vi "MeasureSystemTime.vi"(8 "error in":errorcluster, 11 "VISA resource name":refnum<visa-resource-name>) -> (0 "error out":errorcluster, 1 "System time end":dbl=437416.625 format="%.3f", 2 "System time start":dbl=437416.625 format="%.3f", 3 "VISA resource name out":refnum<visa-resource-name>)   [LabVIEW 2018, in "GP22_TDC_Arduinoed.lvlib"]
doc: "Gets the system time at the start and end of comms. For use in clock sync via NTP-style algorithm."
uses:
  GP22_TDC_Arduinoed.lvlib
  <vilib>/regexp/Match Regular Expression.xnode
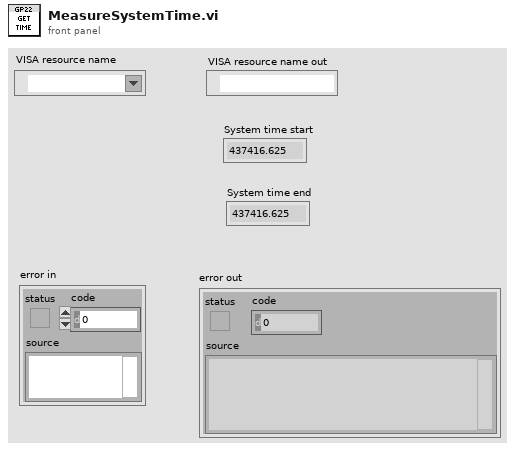
[diagram p1: front panel]
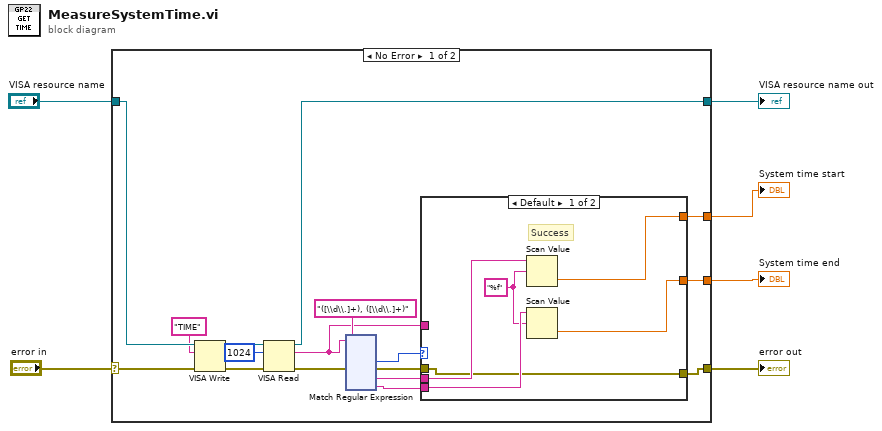
[diagram p0: block diagram]
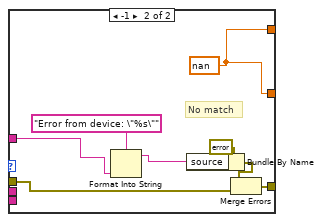
[diagram p2: hidden frame]
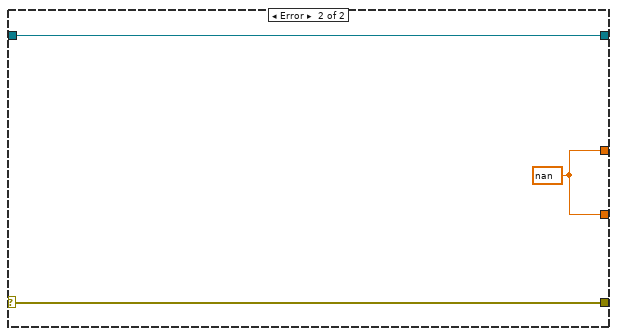
[diagram p3: hidden frame]
diagram:
  n1 = case shown="No Error" "error in" {
    selector: "error in" -> [w23 w157]
    tunnel: [w11 w157] -> w5
    tunnel: [w16 w156] -> w4
    tunnel: "VISA resource name" -> [w22 w156]
    tunnel: [w8 w155] -> w2
    tunnel: [w7 w155] -> w1
    frame No Error {
      n2 = VISA Write(VISA resource name=w22, write buffer="TIME", error in (no error)=w23) -> (VISA resource name out=w19:refnum<visa-resource-name>, error out=w20:errorcluster)  [unwired: 1 out]
      n3 = VISA Read(VISA resource name=w19, byte count=u32 1024, error in (no error)=w20) -> (VISA resource name out=w16:refnum<visa-resource-name>, read buffer=w12:string, error out=w17:errorcluster)  [unwired: 1 out]
      n4 = xnode "Match Regular Expression"("input string"=w12, "regular expression"="([\\d\\.]+), ([\\d\\.]+)", "error in"=w17) -> ("offset past match"=w14:i32, "error out"=w13:errorcluster, "submatch 1"=w10:string, "submatch 2"=w9:string)  [unwired: 3 in, 3 out]
      n5 = case shown="Default" w14 {
        tunnel: w13 -> [w25 w34]
        tunnel: w12 -> [_ w33]
        tunnel: [w25 w36] -> w11
        tunnel: w10 -> [w27 _]
        tunnel: w9 -> [w26 _]
        tunnel: [w29 w30] -> w8
        tunnel: [w28 w30] -> w7
        frame Default {
          w24 = "%f"
          # "Success"
          n6 = Scan Value(string=w27, format string=w24) -> (value=w29:dbl)  [unwired: 1 in, 1 out]
          n7 = Scan Value(string=w26, format string=w24) -> (value=w28:dbl)  [unwired: 1 in, 1 out]
        }
        frame -1 {
          w30 = nan
          # "No match"
          n8 = Format Into String(format string="Error from device: \"%s\"", w33) -> (resulting string=w31:string)  [unwired: 2 in, 1 out]
          n9 = Bundle By Name(cluster=errorcluster {"status"=TRUE, "code"=5000, "source"=""} ("error constant"), "source"=w31) -> (w35:errorcluster)
          n10 = Merge Errors(w35, w34) -> (w36:errorcluster)
        }
      }
    }
    frame Error {
      w155 = nan
    }
  }
  "VISA resource name out" <- w4
  "error out" <- w5
  "System time start" <- w2
  "System time end" <- w1
